vi "PH_BeamlineInformation.ProcCases.vi"(0 "i ref in":refnum<vi>, 1 "selector":string, 2 "Data":T1, 3 "call cluster":T2={"Object"="", "Selector"="", "CallType"=enum."synchronous", "Async Object"="", "Async Selector"="", "Data Descriptor"="", "Data"=[], "Error #"=0, "Expire"=0}, 5 "error in (no error)":errorcluster) -> (14 "i ref out":refnum<vi>, 17 "answer cluster":T2={"Object"="", "Selector"="", "CallType"=enum."synchronous", "Async Object"="", "Async Selector"="", "Data Descriptor"="", "Data"=[], "Error #"=0, "Expire"=0}, 19 "error out":errorcluster)   [LabVIEW 2014, in "PH_BeamlineInformation.lvlib"]
doc: "This method is called by a process from within the default case in the event loop. The methods of a class that are linked to events will be called from THIS method. Add your code here."
uses:
  PH_BeamlineInformation.lvlib
  CSCore/CSSystem/CoreDefs/CoreDefs.call_type.ctl
  CSCore/BaseProcess/BaseProcess.descriptor string definition.ctl
  CSCore/CSSystem/CoreDefs/CoreDefs.rawDataType.ctl
  CSCore/CSSystem/CoreLib/CoreLib.string 2 byte array.vi
  CSCore/BaseProcess/BaseProcess.lvlib
  CSCore/CAEObj/CAEObj.lvlib
  CSCore/CSSystem/CoreLib/CoreLib.lvlib
  PH_SystemInformation/PH_SystemInformation.lvlib
  PH_Common/PH_Common.lvlib
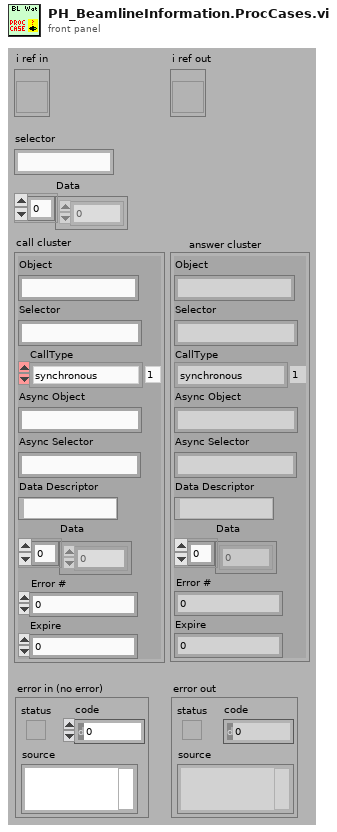
[diagram p1: front panel]
types:
  T1 = typedef "CoreDefs.rawDataType.ctl" = i8[]
  T2 = typedef "CoreDefs.call_type.ctl" = cluster{"Object":string, "Selector":string, "CallType":enum16{"simple", "synchronous", "asynchronous"}, "Async Object":string, "Async Selector":string, "Data Descriptor":T3, "Data":T1, "Error #":i32, "Expire":u32}
  T3 = typedef "BaseProcess.lvlib/BaseProcess.descriptor string definition.ctl" = string
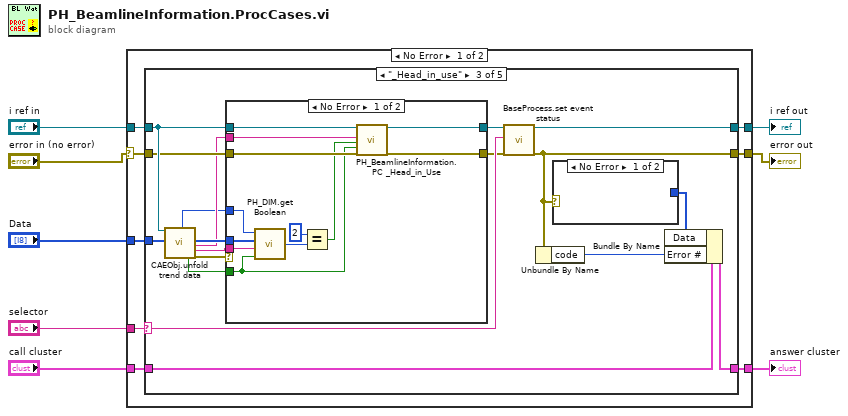
[diagram p0: block diagram]
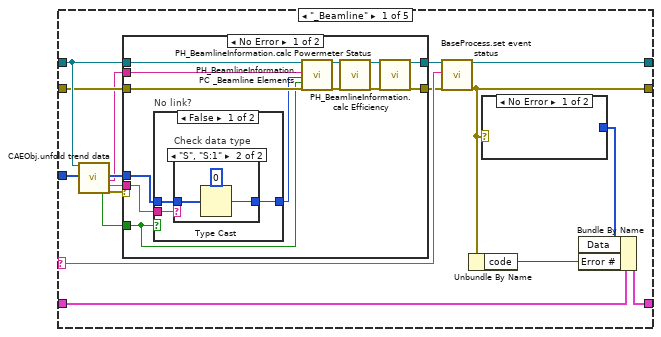
[diagram p2: hidden frame]
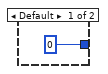
[diagram p3: hidden frame]
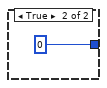
[diagram p4: hidden frame]
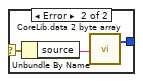
[diagram p6: hidden frame]
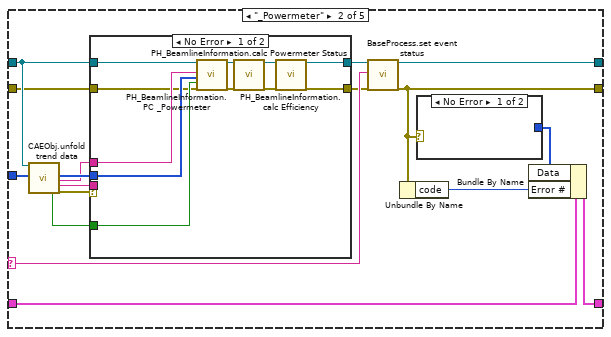
[diagram p7: hidden frame]
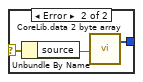
[diagram p9: hidden frame]
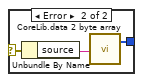
[diagram p11: hidden frame]
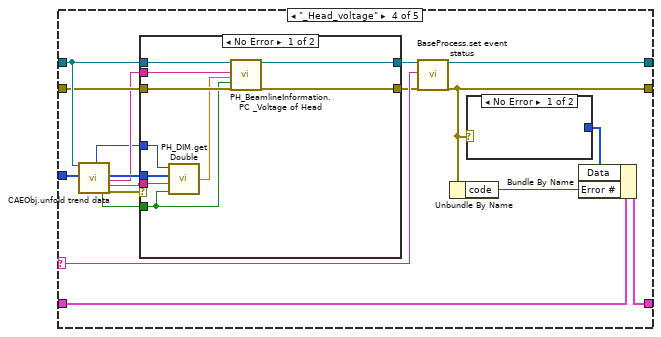
[diagram p12: hidden frame]
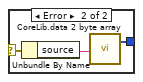
[diagram p14: hidden frame]
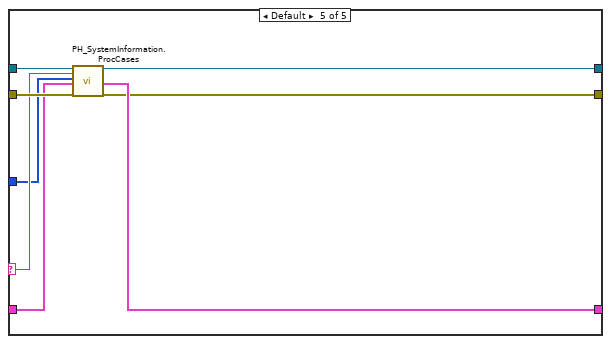
[diagram p15: hidden frame]
diagram:
  n1 = case shown="No Error" "error in (no error)" {
    selector: "error in (no error)" -> [w9 w171]
    tunnel: "selector" -> [w16 _]
    tunnel: [w15 w169] -> w7
    tunnel: "call cluster" -> [w14 w169]
    tunnel: "i ref in" -> [w13 w170]
    tunnel: [w12 w170] -> w4
    tunnel: [w11 w171] -> w3
    tunnel: "Data" -> [w10 _]
    frame No Error {
      n2 = case shown="\"_Head_in_use\"" w16 {
        selector: w16 -> [w29 w72 w106 w141 w165]
        tunnel: w13 -> [w25 w68 w102 w137 w164]
        tunnel: [w31 w74 w108 w143 w162] -> w12
        tunnel: w14 -> [w27 w70 w104 w139 w166]
        tunnel: [w28 w71 w105 w140 w167] -> w15
        tunnel: w9 -> [w23 w66 w100 w135 w168]
        tunnel: [w30 w73 w107 w142 w161] -> w11
        tunnel: w10 -> [w26 w69 w103 w138 w163]
        frame "_Beamline" {
          n3 = call "CAEObj.unfold trend data.vi"("i ref in"=w25, "raw trend data"=w26) -> ("no link"=w18:bool, "data"=w21:i8[], "serviceName"=w17:string, "typeDescriptor"=w19:string, "error out"=w20:errorcluster)  [unwired: 9 in, 4 out]
          n4 = case shown="No Error" w20 {
            tunnel: [w35 w56] -> w24
            tunnel: w25 -> [w46 w56]
            tunnel: w23 -> [w45 w55]
            tunnel: [w34 w55] -> w22
            tunnel: w18 -> [w41 _]
            tunnel: w21 -> [w42 _]
            tunnel: w19 -> [w43 _]
            tunnel: w17 -> [w40 _]
            frame No Error {
              n5 = case "No link?" shown="False" w41 {
                tunnel: [w49 i16 0] -> w44
                tunnel: w42 -> [w48 _]
                tunnel: w43 -> [w47 _]
                frame False {
                  n6 = case "Check data type" shown="\"S\", \"S:1\"" w47 {
                    tunnel: [i16 0 w51] -> w49
                    tunnel: w48 -> [_ w52]
                    frame Default {
                    }
                    frame "S", "S:1" {
                      n7 = Type Cast(type=i16 0, x=w52) -> (*(type *) &x=w51:i16)
                    }
                  }
                }
                frame True {
                }
              }
              n8 = call "PH_BeamlineInformation.PC _Beamline Elements.vi"("i ref in"=w46, "serviceName"=w40, "State"=w44, "not linked?"=w41, "error in (no error)"=w45) -> ("i ref out"=w38:refnum<vi>, "error out"=w39:errorcluster)  [unwired: 13 in]
              n9 = call "PH_BeamlineInformation.calc Powermeter Status.vi"("i ref in"=w38, "error IO"=w39) -> ("i ref out"=w37:refnum<vi>, "error out"=w36:errorcluster)  [unwired: 16 in]
              n10 = call "PH_BeamlineInformation.calc Efficiency.vi"("i ref in"=w37, "error IO"=w36) -> ("i ref out"=w35:refnum<vi>, "error out"=w34:errorcluster)  [unwired: 16 in]
            }
            frame Error {
            }
          }
          n11 = call "BaseProcess.set event status.vi"("i ref in"=w24, "EventStatus"=w29, "error in (no error)"=w22) -> ("i ref out"=w31:refnum<vi>, "error out"=w30:errorcluster)  [unwired: 14 in, 1 out]
          n12 = Unbundle By Name(w30) -> ("code"=w33:i32)
          n13 = case shown="No Error" w30 {
            selector: w30 -> [_ w59]
            tunnel: [_ w57] -> w32
            frame No Error {
            }
            frame Error {
              n14 = Unbundle By Name(w59) -> ("source"=w58:string)
              n15 = call-poly "CoreLib.data 2 byte array.vi"("string"=w58) -> ("byteArray out"=w57:T1)  [unwired: 18 in]
            }
          }
          n16 = Bundle By Name(cluster=w27, "Data"=w32, "Error #"=w33) -> (w28:T2)
        }
        frame "_Powermeter" {
          n17 = call "CAEObj.unfold trend data.vi"("i ref in"=w68, "raw trend data"=w69) -> ("no link"=w61:bool, "data"=w64:i8[], "serviceName"=w60:string, "typeDescriptor"=w62:string, "error out"=w63:errorcluster)  [unwired: 9 in, 4 out]
          n18 = case shown="No Error" w63 {
            tunnel: [w83 w89] -> w67
            tunnel: w68 -> [w82 w89]
            tunnel: w66 -> [w81 w88]
            tunnel: [w84 w88] -> w65
            tunnel: w61 -> [w87 _]
            tunnel: w64 -> [w85 _]
            tunnel: w62 -> [_ _]
            tunnel: w60 -> [w86 _]
            frame No Error {
              n19 = call "PH_BeamlineInformation.PC _Powermeter.vi"("i ref in"=w82, "serviceName"=w86, "data"=w85, "not linked?"=w87, "error in (no error)"=w81) -> ("i ref out"=w78:refnum<vi>, "error out"=w80:errorcluster)  [unwired: 13 in]
              n20 = call "PH_BeamlineInformation.calc Powermeter Status.vi"("i ref in"=w78, "error IO"=w80) -> ("i ref out"=w77:refnum<vi>, "error out"=w79:errorcluster)  [unwired: 16 in]
              n21 = call "PH_BeamlineInformation.calc Efficiency.vi"("i ref in"=w77, "error IO"=w79) -> ("i ref out"=w83:refnum<vi>, "error out"=w84:errorcluster)  [unwired: 16 in]
            }
            frame Error {
            }
          }
          n22 = call "BaseProcess.set event status.vi"("i ref in"=w67, "EventStatus"=w72, "error in (no error)"=w65) -> ("i ref out"=w74:refnum<vi>, "error out"=w73:errorcluster)  [unwired: 14 in, 1 out]
          n23 = Unbundle By Name(w73) -> ("code"=w76:i32)
          n24 = case shown="No Error" w73 {
            selector: w73 -> [_ w92]
            tunnel: [_ w90] -> w75
            frame No Error {
            }
            frame Error {
              n25 = Unbundle By Name(w92) -> ("source"=w91:string)
              n26 = call-poly "CoreLib.data 2 byte array.vi"("string"=w91) -> ("byteArray out"=w90:T1)  [unwired: 18 in]
            }
          }
          n27 = Bundle By Name(cluster=w70, "Data"=w75, "Error #"=w76) -> (w71:T2)
        }
        frame "_Head_in_use" {
          n28 = call "CAEObj.unfold trend data.vi"("i ref in"=w102, "raw trend data"=w103) -> ("quality"=w93:i32, "no link"=w95:bool, "data"=w98:i8[], "serviceName"=w94:string, "typeDescriptor"=w96:string, "error out"=w97:errorcluster)  [unwired: 9 in, 3 out]
          n29 = case shown="No Error" w97 {
            tunnel: [w116 w124] -> w101
            tunnel: w102 -> [w117 w124]
            tunnel: w100 -> [w119 w123]
            tunnel: [w118 w123] -> w99
            tunnel: w95 -> [w114 _]
            tunnel: w98 -> [w121 _]
            tunnel: w96 -> [w122 _]
            tunnel: w94 -> [w115 _]
            tunnel: w93 -> [w120 _]
            frame No Error {
              n30 = call "PH_DIM.get Boolean.vi"("no link"=w114, "typeDescriptor"=w122, "data"=w121, "quality"=w120) -> ("Value"=w113:i32)
              n31 = Equal?(x=2, y=w113) -> (x = y?=w112:bool)
              n32 = call "PH_BeamlineInformation.PC _Head_in_Use.vi"("i ref in"=w117, "In Use Service Name"=w115, "In Use?"=w112, "no link?"=w114, "error in (no error)"=w119) -> ("i ref out"=w116:refnum<vi>, "error out"=w118:errorcluster)  [unwired: 13 in]
            }
            frame Error {
            }
          }
          n33 = call "BaseProcess.set event status.vi"("i ref in"=w101, "EventStatus"=w106, "error in (no error)"=w99) -> ("i ref out"=w108:refnum<vi>, "error out"=w107:errorcluster)  [unwired: 14 in, 1 out]
          n34 = Unbundle By Name(w107) -> ("code"=w110:i32)
          n35 = case shown="No Error" w107 {
            selector: w107 -> [_ w127]
            tunnel: [_ w125] -> w109
            frame No Error {
            }
            frame Error {
              n36 = Unbundle By Name(w127) -> ("source"=w126:string)
              n37 = call-poly "CoreLib.data 2 byte array.vi"("string"=w126) -> ("byteArray out"=w125:T1)  [unwired: 18 in]
            }
          }
          n38 = Bundle By Name(cluster=w104, "Data"=w109, "Error #"=w110) -> (w105:T2)
        }
        frame "_Head_voltage" {
          n39 = call "CAEObj.unfold trend data.vi"("i ref in"=w137, "raw trend data"=w138) -> ("quality"=w128:i32, "no link"=w130:bool, "data"=w133:i8[], "serviceName"=w129:string, "typeDescriptor"=w131:string, "error out"=w132:errorcluster)  [unwired: 9 in, 3 out]
          n40 = case shown="No Error" w132 {
            tunnel: [w149 w157] -> w136
            tunnel: w137 -> [w150 w157]
            tunnel: w135 -> [w152 w156]
            tunnel: [w151 w156] -> w134
            tunnel: w130 -> [w148 _]
            tunnel: w133 -> [w154 _]
            tunnel: w131 -> [w155 _]
            tunnel: w129 -> [w147 _]
            tunnel: w128 -> [w153 _]
            frame No Error {
              n41 = call "PH_DIM.get Double.vi"("no link"=w148, "typeDescriptor"=w155, "data"=w154, "quality"=w153) -> ("Value"=w146:dbl)
              n42 = call "PH_BeamlineInformation.PC _Voltage of Head.vi"("i ref in"=w150, "Voltage Service Name"=w147, "Voltage [V]"=w146, "no link?"=w148, "error in (no error)"=w152) -> ("i ref out"=w149:refnum<vi>, "error out"=w151:errorcluster)  [unwired: 13 in]
            }
            frame Error {
            }
          }
          n43 = call "BaseProcess.set event status.vi"("i ref in"=w136, "EventStatus"=w141, "error in (no error)"=w134) -> ("i ref out"=w143:refnum<vi>, "error out"=w142:errorcluster)  [unwired: 14 in, 1 out]
          n44 = Unbundle By Name(w142) -> ("code"=w145:i32)
          n45 = case shown="No Error" w142 {
            selector: w142 -> [_ w160]
            tunnel: [_ w158] -> w144
            frame No Error {
            }
            frame Error {
              n46 = Unbundle By Name(w160) -> ("source"=w159:string)
              n47 = call-poly "CoreLib.data 2 byte array.vi"("string"=w159) -> ("byteArray out"=w158:T1)  [unwired: 18 in]
            }
          }
          n48 = Bundle By Name(cluster=w139, "Data"=w144, "Error #"=w145) -> (w140:T2)
        }
        frame Default {
          # "In the default case, always call the ProcCase method of the parent class"
          n49 = call "PH_SystemInformation.ProcCases.vi"("i ref in"=w164, "selector"=w165, "Data"=w163, "call cluster"=w166, "error in (no error)"=w168) -> ("i ref out"=w162:refnum<vi>, "answer cluster"=w167:T2, "error out"=w161:errorcluster)  [unwired: 12 in]
        }
      }
    }
    frame Error {
    }
  }
  "answer cluster" <- w7
  "i ref out" <- w4
  "error out" <- w3
